vi "Read DBC Subfunction.vi"(8 "error In":errorcluster, 11 "Frames":refnum<k21>[](array[refnum])) -> (0 "error out":errorcluster, 3 "Sigs":refnum<k21>[](array[refnum]))   [LabVIEW 2018]
uses:
  <resource>/objmgr/xnet.rc
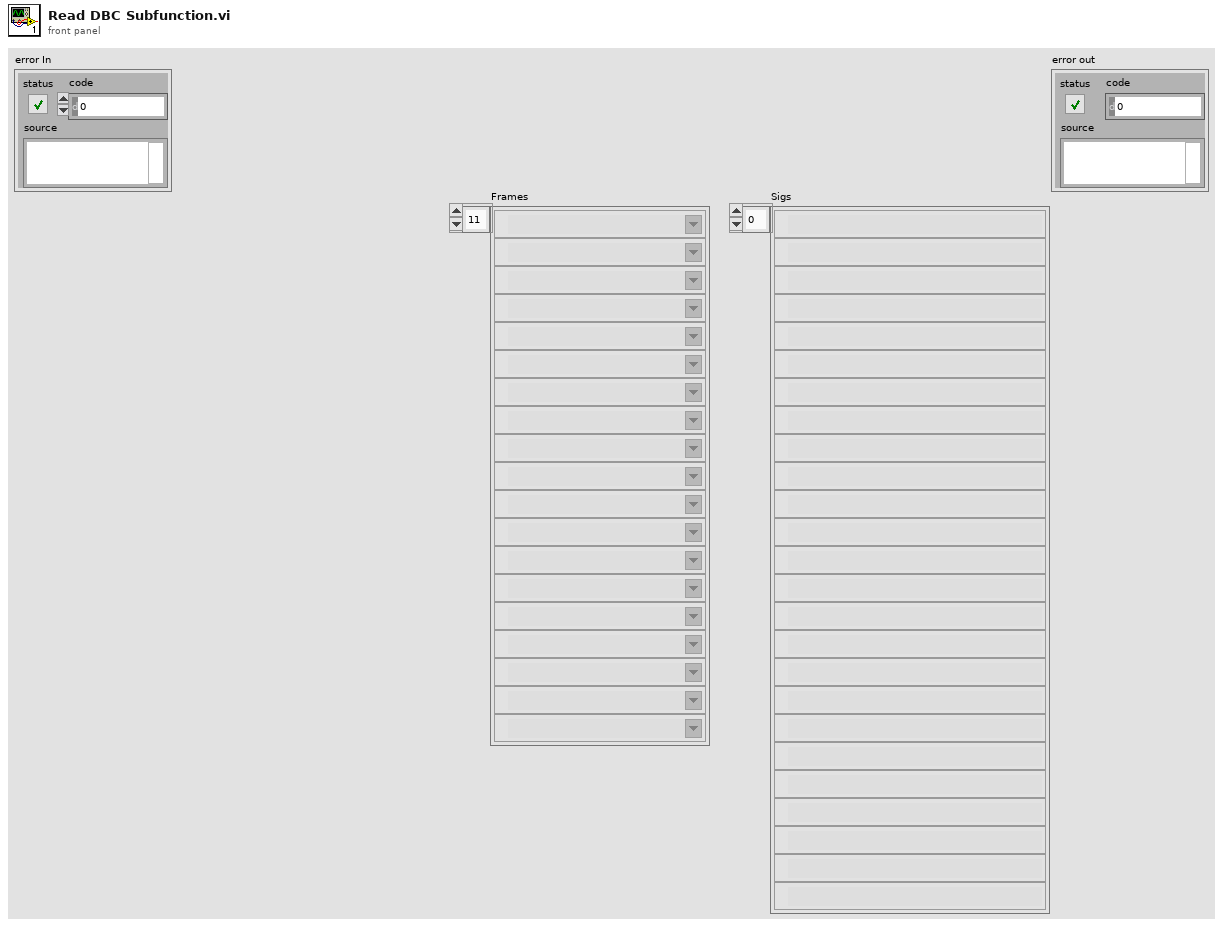
[diagram p1: front panel]
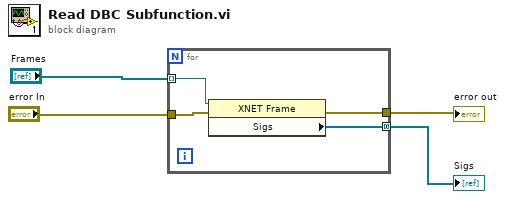
[diagram p0: block diagram]
diagram:
  n1 = for {
    tunnel: "Frames" -> [w8] mode=indexing
    tunnel: [w7] -> w3 mode=concatenating
    tunnel: "error In" -> [w6]
    tunnel: [w5] -> w1
    n2 = property class="XNET Frame"(reference=w8, error in=w6) -> (error out=w5:errorcluster, "Sigs"=w7:refnum<k21>[])  [unwired: 1 out]
  }
  "Sigs" <- w3
  "error out" <- w1
